vi "Write Packet Type.vi"(8 "error in (no error)":errorcluster, 10 "Packet Type":string, 11 "JSONPayload in":refnum<class "JSONPayload.lvclass">) -> (0 "error out":errorcluster, 3 "JSONPayload out":refnum<class "JSONPayload.lvclass">)   [LabVIEW 2019, in "JSONPayload.lvclass"]
uses:
  JSONPayload.lvclass
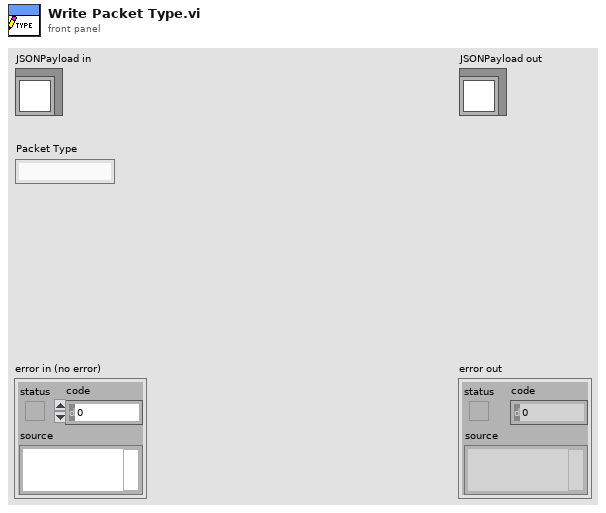
[diagram p1: front panel]
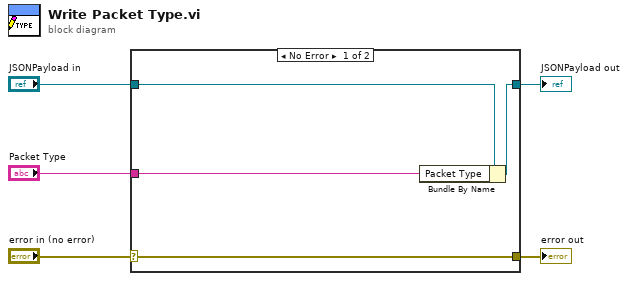
[diagram p0: block diagram]
diagram:
  n1 = case shown="No Error" "error in (no error)" {
    selector: "error in (no error)" -> [w9 w10]
    tunnel: [w9 w10] -> w4
    tunnel: [w7 w11] -> w2
    tunnel: "JSONPayload in" -> [w8 w11]
    tunnel: "Packet Type" -> [w6 _]
    frame No Error {
      n2 = Bundle By Name(cluster=w8, "Packet Type"=w6) -> (w7:refnum<class "JSONPayload.lvclass">)
    }
    frame Error {
    }
  }
  "error out" <- w4
  "JSONPayload out" <- w2
